vi "O3manifold.vi"(7 "LabVIEW Web Service Request":refnum<class "Web Request.lvclass">, 11 "On":u8) -> ()   [LabVIEW 2014]
uses:
  <vilib>/wsapi/Web Request.lvclass
  <vilib>/DAQmx/write.llb/DAQmx Write (Digital Bool 1Line 1Point).vi
panel:
  # "Use the Web Service Request input terminal to call the VIs on the Web Services palette. Do not remove it from the connector pane unless you don't need access to the palette."
  # "Each additional control wired to the connector pane will be available as an input in the URL. To include an indicator in terminal-mode output (the default setting), it must also be wired to the connector pane."
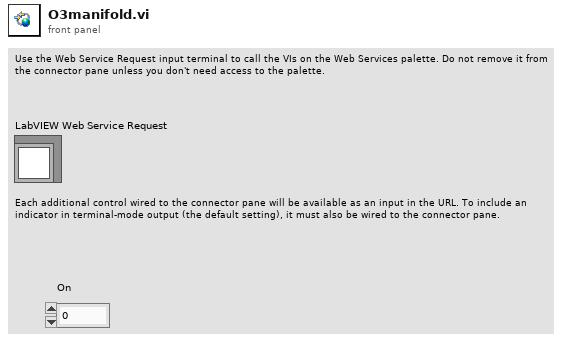
[diagram p1: front panel]
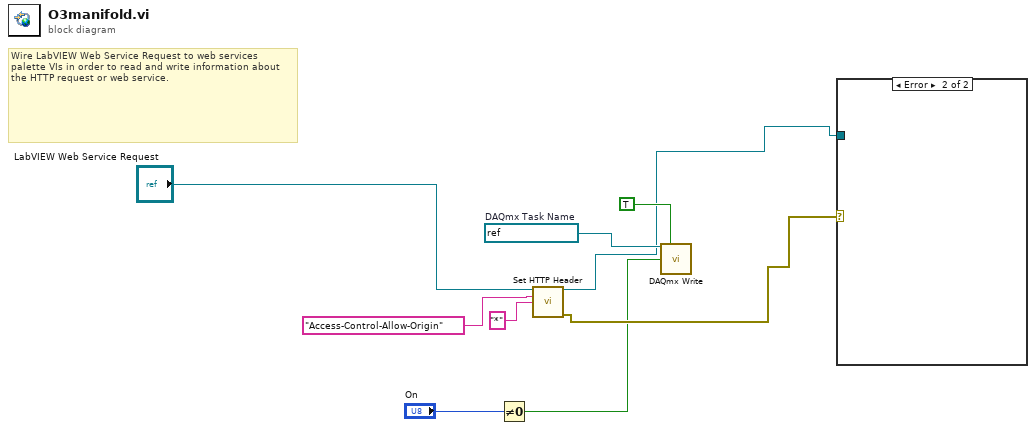
[diagram p0: block diagram]
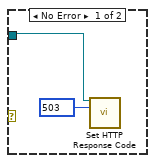
[diagram p2: hidden frame]
diagram:
  w6 = refnum<k21> "O3 manifold"  # DAQmx Task Name
  # "Wire LabVIEW Web Service Request to web services palette VIs in order to read and write information about the HTTP request or web service."
  n1 = Not Equal To 0?(x="On") -> (x != 0?=w1:bool)
  n2 = call <vilib>:"Set HTTP Header.vi"("LabVIEW Web Service Request"="LabVIEW Web Service Request", "header"="Access-Control-Allow-Origin", "header value"="*") -> ("LabVIEW Web Service Request out"=w2:refnum<class "Web Request.lvclass">, "error out"=w3:errorcluster)  [unwired: 11 in]
  n3 = call-poly <vilib>:"DAQmx Write.vi"("task/channels in"=w6, "auto start"=TRUE, "data"=w1) -> ()  [unwired: 10 in, 3 out]
  n4 = case shown="Error" w3 {
    tunnel: w2 -> [w10 _]
    frame No Error {
      w11 = 503 items=["100"=100, "101"=101, "200"=200, "201"=201, "202"=202, "203"=203, "204"=204, "205"=205, "206"=206, "300"=300, "301"=301, "302"=302, "303"=303, "304"=304, "305"=305, "306"=306, "307"=307, "400"=400, "401"=401, "402"=402, "403"=403, "404"=404, "405"=405, "406"=406, "407"=407, "408"=408, "409"=409, "410"=410, "411"=411, "412"=412, "413"=413, "414"=414, "415"=415, "416"=416, "417"=417, "500"=500, "501"=501, "502"=502, "503"=503, "504"=504, "505"=505] ("response code (200)")
      n5 = call <vilib>:"Set HTTP Response Code.vi"("LabVIEW Web Service Request"=w10, "response code (200)"=w11) -> ()  [unwired: 12 in, 2 out]
    }
    frame Error {
    }
  }
